vi "Comprar Message.vi"(8 "error in (no error)":errorcluster, 11 "Mensajes in":refnum<class "Mensajes.lvclass">) -> (0 "error out":errorcluster, 3 "Mensajes out":refnum<class "Mensajes.lvclass">)   [LabVIEW 2020, in "Mensajes.lvlib" / "Mensajes.lvclass"]
uses:
  Mensajes.lvclass
  C:/Program Files (x86)/National Instruments/LabVIEW 2020/vi.lib/ActorFramework/Actor/Actor.lvclass
  <vilib>/ActorFramework/Actor/Actor.lvclass/Actor.ctl
  Mensajes.lvclass/Mensajes.ctl
  <vilib>/ActorFramework/Message Enqueuer/Message Enqueuer.lvclass/Message Enqueuer.ctl
  User Interface Messages/Update credit Msg/Update credit Msg.lvclass/Update credit Msg.ctl
  <vilib>/ActorFramework/Message Enqueuer/Enqueue.vi
  User Interface Messages/Update producto Msg/Update producto Msg.lvclass
  C:/Program Files (x86)/National Instruments/LabVIEW 2020/vi.lib/ActorFramework/Message/Message.lvclass
  User Interface Messages/Update credit Msg/Update credit Msg.lvclass
  <vilib>/ActorFramework/Message Priority Queue/Priority Enqueue.vi
  <vilib>/ActorFramework/Actor/Actor.lvclass
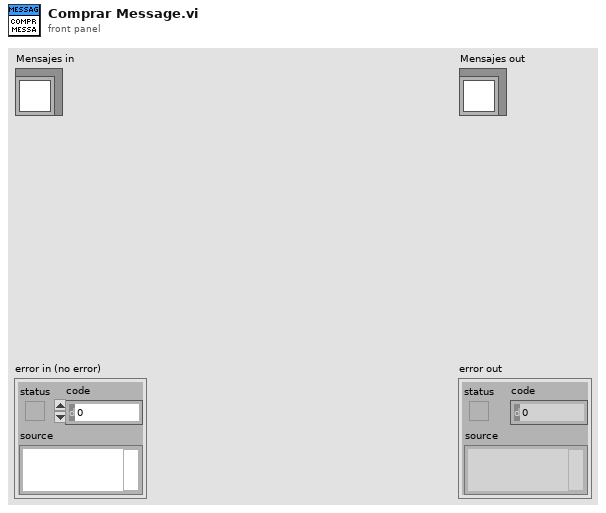
[diagram p1: front panel]
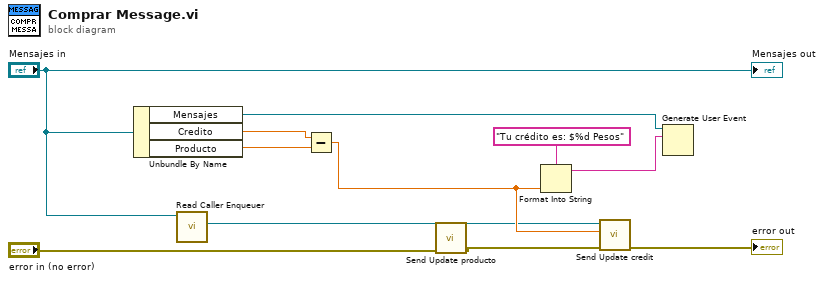
[diagram p0: block diagram]
diagram:
  n1 = Unbundle By Name("Mensajes in") -> ("Mensajes"=w12:refnum<user-event>, "Credito"=w9:dbl, "Producto"=w8:dbl)
  n2 = call <vilib>:"Read Caller Enqueuer.vi"("Actor"="Mensajes in") -> ("Caller Enqueuer"=w2:refnum<class "Message Enqueuer.lvclass">)  [unwired: 10 in]
  n3 = Subtract(x=w9, y=w8) -> (x-y=w6:dbl)
  n4 = call "Send Update producto.vi"("error in (no error)"="error in (no error)", "Message Enqueuer"=w2) -> ("error out"=w4:errorcluster, "Message Enqueuer out"=w1:refnum<class "Message Enqueuer.lvclass">)  [unwired: 8 in]
  n5 = Format Into String(format string="Tu crédito es: $%d Pesos", w6) -> (resulting string=w10:string)  [unwired: 2 in, 1 out]
  n6 = call "Send Update credit.vi"("error in (no error)"=w4, "Credit"=w6, "Message Enqueuer"=w1) -> ("error out"=→"error out":errorcluster)  [unwired: 7 in, 1 out]
  n7 = Generate User Event(user event=w12, event data cluster=w10) -> ()  [unwired: 2 in, 2 out]
  "Mensajes out" <- "Mensajes in"
